vi "Verify With 3 Scrubbers.vi"(11 "LUnit Test Case In":refnum<class "Test Case.lvclass">) -> (0 "error out":errorcluster, 3 "LUnit Test Case Out":refnum<class "Test Case.lvclass">)   [LabVIEW 2020, in "Scrubber Tests.lvclass"]
uses:
  Scrubber Tests.lvclass
  <vilib>/Astemes/LUnit/Test Case.lvclass
  Source/Approval Tests/Options/Options.lvclass
  Source/Approval Tests/Regex Scrubber/Regex Scrubber.lvclass
  C:/Users/SAS/Desktop/ApprovalTests.LabVIEW/Source/Approval Tests/Scrubber/Scrubber.lvclass
  Source/Approval Tests/Regex Scrubber/Regex Scrubber.lvclass/Regex Scrubber.ctl
  Source/Approval Tests/Options/Options.lvclass/Options.ctl
  Source/Approval Tests/Naming Data/Naming Data.lvclass/Naming Data.ctl
  <vilib>/Astemes/LUnit/Test Case.lvclass/Test Case.ctl
  d22741b7-9abc-4f28-b51a-54e5e2d59af2.vi
  Source/Approval Tests/Regex Scrubber/Write Regex.vi
  Source/Approval Tests/Regex Scrubber/Write Replacement.vi
  d22741b7-9abc-4f28-b51a-54e5e2d59af2.vi/1e051690-6811-4db0-8b8f-f6ad9423d026.vi
  Source/Approval Tests/Replace if Empty.vi
  <vilib>/Astemes/LUnit/Palette/Pass If.vi
  Source/Approval Tests/Options/Update Test Name if Not Defined.vi
  Source/Approval Tests/Verify Core.vi
  d22741b7-9abc-4f28-b51a-54e5e2d59af2.vi/1e051690-6811-4db0-8b8f-f6ad9423d026.vi/93c5622b-9fb7-41e0-8c76-3fde37e94e34.vi
  Source/Approval Tests/Options/Read Scrubber.vi
  <vilib>/Astemes/LUnit/Core/LUnit Test Case/Private/Append Fail Result.vi
  <vilib>/Astemes/LUnit/Core/LUnit Test Case/Private/Append Pass Result.vi
  Source/Approval Tests/Naming Data/Read Test VI Name.vi
  Source/Approval Tests/Naming Data/Write Test VI Name.vi
  Source/Approval Tests/Options/Read Namer.vi
  Source/Approval Tests/Options/Read Naming Data.vi
  Source/Approval Tests/Options/Read Reporter.vi
  Source/Approval Tests/Options/Read Text Comparator.vi
  d22741b7-9abc-4f28-b51a-54e5e2d59af2.vi/1e051690-6811-4db0-8b8f-f6ad9423d026.vi/93c5622b-9fb7-41e0-8c76-3fde37e94e34.vi/04cb982b-2eda-40d0-8d7e-90f8e0b569b2.vi
  <vilib>/Astemes/LUnit/Core/LUnit Test Case/Private/Run In UI.vi
  <vilib>/Utility/error.llb/Clear Errors.vi
  Source/Approval Tests/Options/Write Add Scrubber.vi
  Source/Approval Tests/Options/Add Label to Namer.vi
  Source/Approval Tests/conv EOL.vi
  <vilib>/Utility/libraryn.llb/Check if File or Folder Exists.vi
  Source/Approval Tests/Reporter/Report.vi
  Source/Approval Tests/Scrubber/Scrubber.lvclass
  Source/Approval Tests/Namer/Namer.lvclass
  Source/Approval Tests/Naming Data/Naming Data.lvclass
  Source/Approval Tests/Reporter/Reporter.lvclass
  Source/Approval Tests/Text Comparator/Text Comparator.lvclass
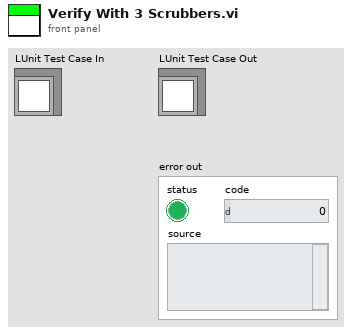
[diagram p1: front panel]
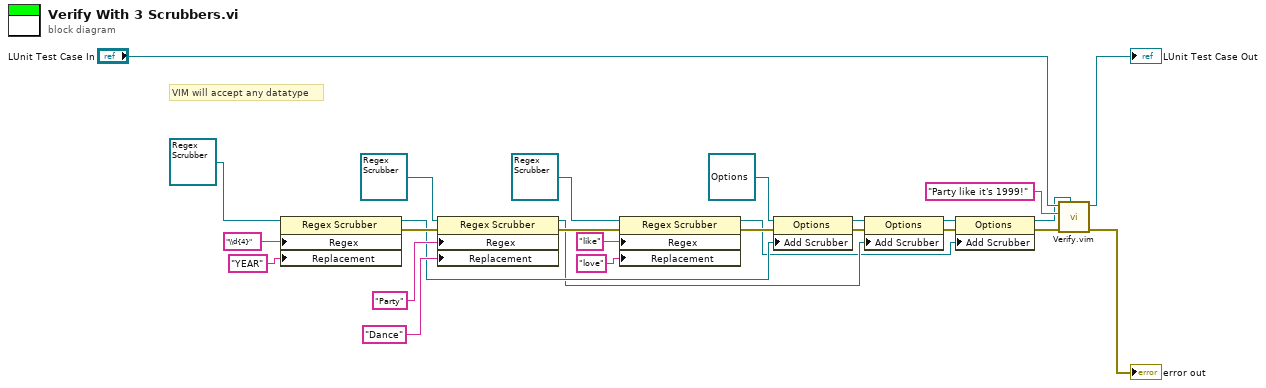
[diagram p0: block diagram]
diagram:
  # "VIM will accept any datatype"
  n1 = property class="Regex Scrubber"(reference=refnum<class "Regex Scrubber.lvclass"> refnum ("Approval Tests.lvlib:Regex Scrubber.lvclass"), "Regex"="\\d{4}", "Replacement"="YEAR") -> (reference out=w12:refnum<class "Regex Scrubber.lvclass">, error out=w26:errorcluster)  [unwired: 1 in]
  n2 = property class="Regex Scrubber"(reference=refnum<class "Regex Scrubber.lvclass"> refnum ("Approval Tests.lvlib:Regex Scrubber.lvclass"), error in=w26, "Regex"="Party", "Replacement"="Dance") -> (reference out=w10:refnum<class "Regex Scrubber.lvclass">, error out=w25:errorcluster)
  n3 = property class="Regex Scrubber"(reference=refnum<class "Regex Scrubber.lvclass"> refnum ("Approval Tests.lvlib:Regex Scrubber.lvclass"), error in=w25, "Regex"="like", "Replacement"="love") -> (reference out=w5:refnum<class "Regex Scrubber.lvclass">, error out=w22:errorcluster)
  n4 = property class="Options"(reference=refnum<class "Options.lvclass"> refnum ("Approval Tests.lvlib:Options.lvclass"), error in=w22, "Add Scrubber"=w12) -> (reference out=w11:refnum<class "Options.lvclass">, error out=w24:errorcluster)
  n5 = property class="Options"(reference=w11, error in=w24, "Add Scrubber"=w10) -> (reference out=w9:refnum<class "Options.lvclass">, error out=w23:errorcluster)
  n6 = property class="Options"(reference=w9, error in=w23, "Add Scrubber"=w5) -> (reference out=w1:refnum<class "Options.lvclass">, error out=w20:errorcluster)
  n7 = call "Verify.vim"("Options"=w1, "error in"=w20, "Test Data"="Party like it's 1999!", "LUnit Test Case In"="LUnit Test Case In") -> ("error out"=→"error out":errorcluster, "LUnit Test Case Out"=→"LUnit Test Case Out":refnum<class "Test Case.lvclass">)  [unwired: 6 in]
